vi "Numeric Control - Radio.vi"() -> ()   [LabVIEW 2015, in "Workspace.Obejct.Radio.lvlib"]
doc: "Sample numeric display item."
uses:
  Workspace.Obejct.Radio.lvlib
  <vilib>/NI Veristand/Display Template Support/Display Template Support.llb/cluster_Screen Item Settings.ctl
  <vilib>/NI Veristand/Display Template Support/Display Template Support.llb/cluster_Graph Scale Settings.ctl
  <vilib>/NI Veristand/Display Template Support/Display Template Support.llb/cluster_Graph Plot Settings.ctl
  NationalInstruments.VeriStand.SystemStorage
  <vilib>/NI Veristand/Display Template Support/Display Template Support.llb/enum_Display Template Handler Minimal To Widget Msg.ctl
  <vilib>/NI Veristand/Display Template Support/Display Template Support.llb/enum_Display Template Handler Minimal To Workspace.ctl
  Types/StateVariables.ctl
  <vilib>/NI Veristand/Execution/Workspace/WorkspaceAPI.ctl
  Types/SavedStateData.ctl
  Types/Config.ctl
  <vilib>/NI Veristand/Execution/Workspace/SystemStateEventRef.ctl
  <vilib>/NI Veristand/Execution/Workspace/Target State Info.ctl
  <vilib>/NI Veristand/Execution/Workspace/Target State.ctl
  <vilib>/NI Veristand/Execution/Workspace/SystemStateRegEventRef.ctl
  <vilib>/NI Veristand/Display Template Support/Display Template Support.llb/sub_Display Template Handler Custom.vi
  <vilib>/NI Veristand/Execution/Workspace/NI VeriStand - Set Single Channel Value.vi
  <vilib>/NI Veristand/Execution/Workspace/NI VeriStand - Get Single Channel Value.vi
  <vilib>/NI Veristand/Execution/Workspace/NI_VS Workspace ExecutionAPI.lvlib
  NationalInstruments.VeriStand.ClientAPI
panel:
  in  "NIVS.Gateway IP Address":string
  in  "Listbox":i32(listbox) caption="Channel"
  in  "NIVS.System Definition Root":refnum<k24>
  in  "Item.Data":T1
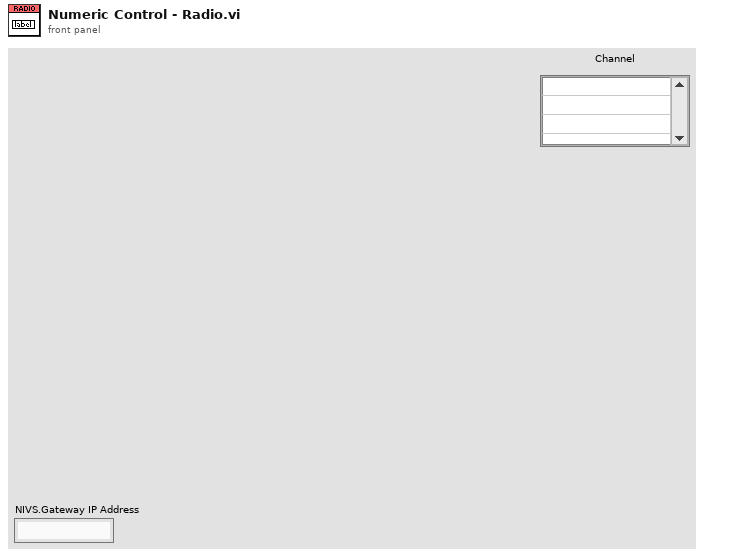
[diagram p1: front panel]
types:
  T1 = typedef "cluster_Screen Item Settings.ctl" = cluster{"Template VI":string, "Position X":i32, "Position Y":i32, "Custom":string, "Show Title Bar":bool, "ID":i32, "Always On Top":bool, "Allow Resize":bool, "Allow Minimize":bool, "Allow Close":bool, "Size to Screen":bool, "Screen.ID":i32, "State":enum16{"Normal", "New"}, "Title":string, "Window Bounds":cluster{"[0]":i16, "[1]":i16, "[2]":i16, "[3]":i16}, "Channel Ref":u64, "Unit":string, "Default Units?":bool, "Flash Limit?":bool, "Color 1":u32, "Color 2":u32, "Color 3":u32, "Color 4":u32, "Bck Color":u32, "Fore Color":u32, "Limit 1":dbl, "Limit 2":dbl, "Limit 3":dbl, "Limit 4":dbl, "Limit Mode 1":i32, "Limit Mode 2":i32, "Limit Mode 3":i32, "Limit Mode 4":i32, "Scale Precision":i32, "Scale Min":dbl, "Scale Max":dbl, "Format":i32, "Precision":i32, "Background Type":i32, "IDs":i32[], "Units":string[], "Labels":string[], "Scale Factor":dbl, "Scale Offset":dbl, "YScale Index":u32[], "XScale":T2, "YScales":T2[], "Plots":T3[], "Update Period":dbl, "History Length":dbl, "My.Ref":refnum<vi>, "Is Control?":bool, "Channel Paths":string[], "Custom Data":variant}
  T2 = typedef "cluster_Graph Scale Settings.ctl" = cluster{"Format":u8, "Precision":u8, "Fit":u8, "Label":string, "Use Default Label":bool, "Label Visible":bool, "Min":dbl, "Max":dbl}
  T3 = typedef "cluster_Graph Plot Settings.ctl" = cluster{"Bar Style":u8, "Fill To":i16, "Fill/PtColor":u32, "Line Style":u8, "Line Width":u8, "Color":u32, "Interp":u8, "Point Style":u8}
  T4 = typedef "Workspace.Obejct.Radio.lvlib/StateVariables.ctl" = cluster{"NIVS.CachedDataRef":refnum<user-event>, "NIVS.LaunchRef":refnum<user-event>, "NIVS.SysDefRoot":refnum<k24>, "NIVS.Workspace":T5, "NIVS.CachedData":T6, "NIVS.SystemStateRefs":T8, "NIVS.UserEventRefs":cluster{"SystemChangeEventRef":T9, "Event Registration Refnum":refnum<event-registration>}, "Workspace.Connected?":bool, "Workspace.ChannelFound?":bool, "UI.Listbox":refnum<vi>, "VS.DisplayFilter":u8, "Force?":bool}
  T5 = typedef "NI_VS Workspace ExecutionAPI.lvlib/WorkspaceAPI.ctl" = refnum<k24>
  T6 = typedef "Workspace.Obejct.Radio.lvlib/SavedStateData.ctl" = cluster{"Name":string, "Node Path":string, "Caption":string, "List":T7}
  T7 = typedef "Workspace.Obejct.Radio.lvlib/Config.ctl" = cluster{"AutoUpdate":bool, "Names":string[], "Values":dbl[], "Symbols":i32[]}
  T8 = typedef "NI_VS Workspace ExecutionAPI.lvlib/SystemStateEventRef.ctl" = cluster{"CustDatRef":refnum<user-event>, "EvtRef":refnum<k27>, "Target State User Event":refnum<user-event>}
  T9 = typedef "NI_VS Workspace ExecutionAPI.lvlib/SystemStateRegEventRef.ctl" = refnum<event-registration>
  T10 = typedef "enum_Display Template Handler Minimal To Workspace.ctl" = cluster{"Operation":enum16{"SetCustomData", "DeleteItem"}, "Data":variant}
  T11 = typedef "enum_Display Template Handler Minimal To Widget Msg.ctl" = enum16{"Stop", "LaunchConfigDialog"}
  T12 = typedef "NI_VS Workspace ExecutionAPI.lvlib/SystemState.ctl" = u8
  T13 = cluster{"SystemChangeEventRef":T9, "Event Registration Refnum":refnum<event-registration>}
  T14 = typedef "NI_VS UI Single Node Browser.lvlib/Node Ref.ctl" = refnum<k24>
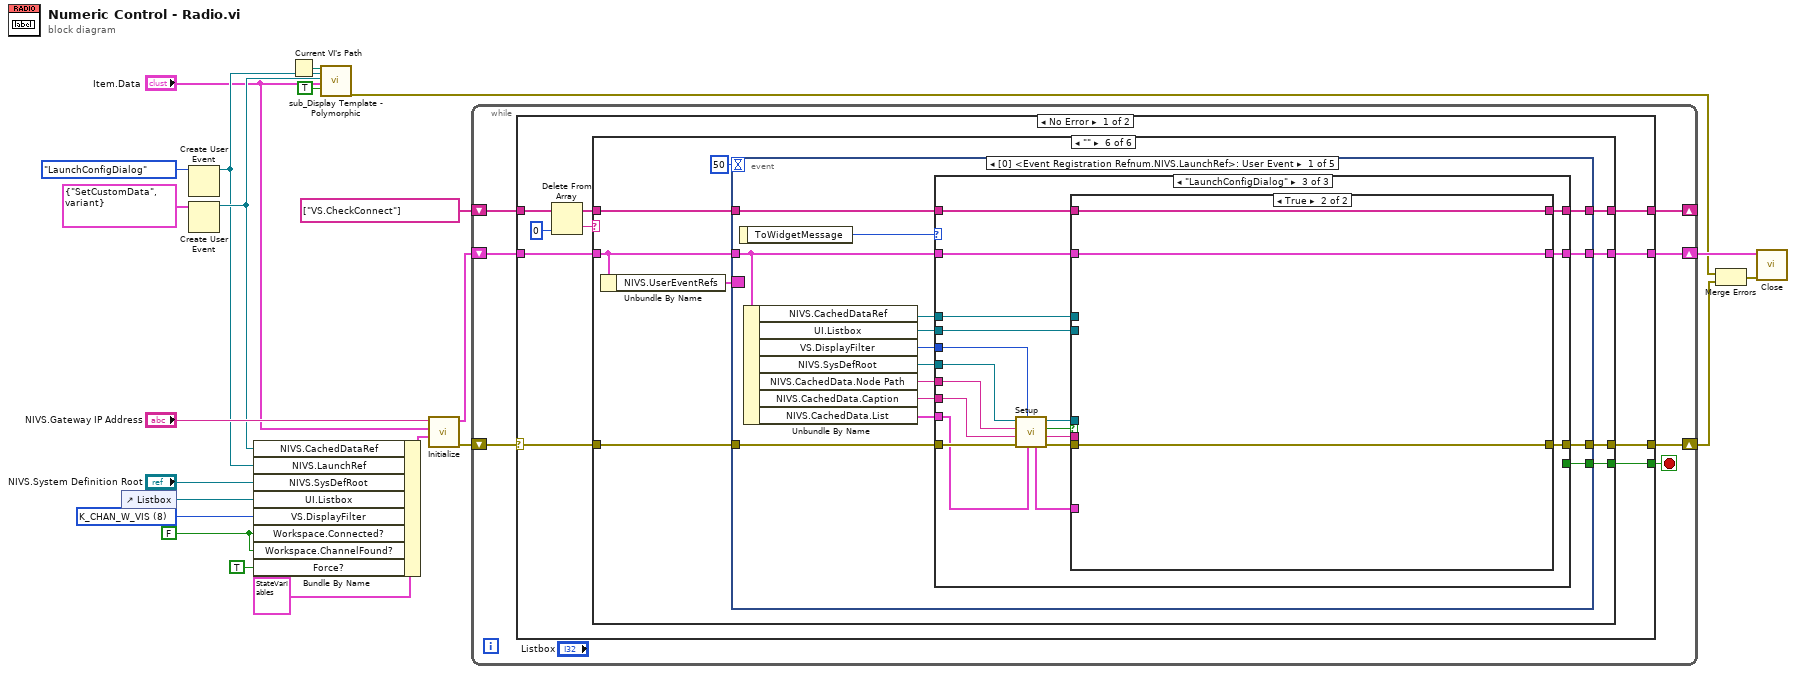
[diagram p0: block diagram]
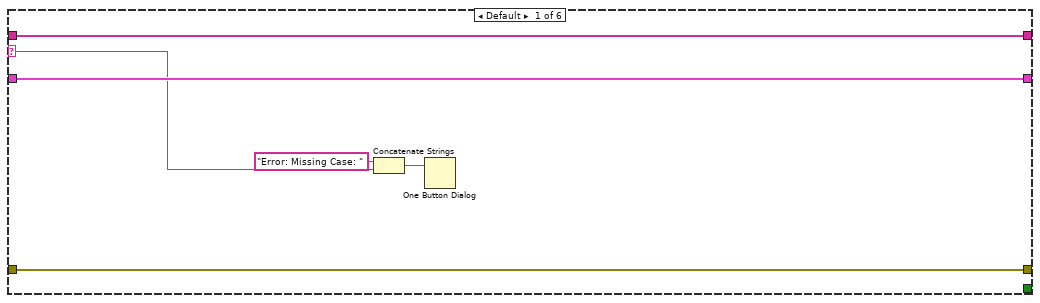
[diagram p2: hidden frame]
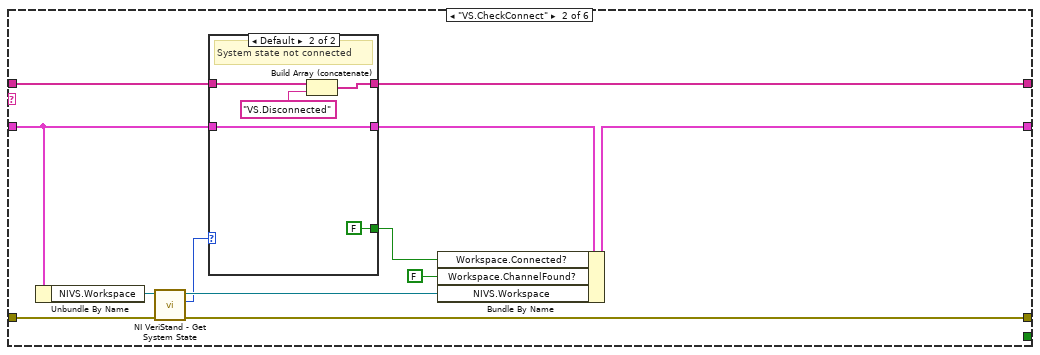
[diagram p3: hidden frame]
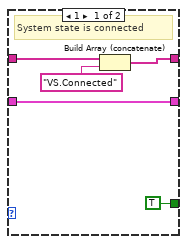
[diagram p4: hidden frame]
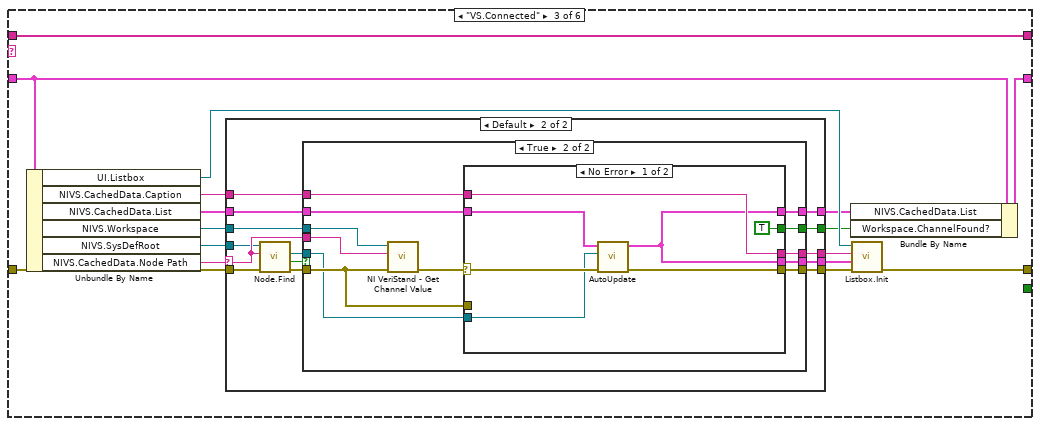
[diagram p5: hidden frame]
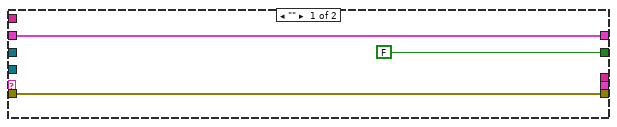
[diagram p6: hidden frame]
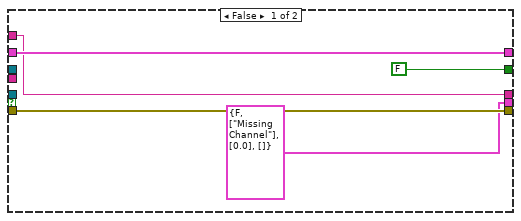
[diagram p7: hidden frame]
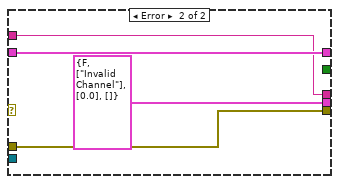
[diagram p8: hidden frame]
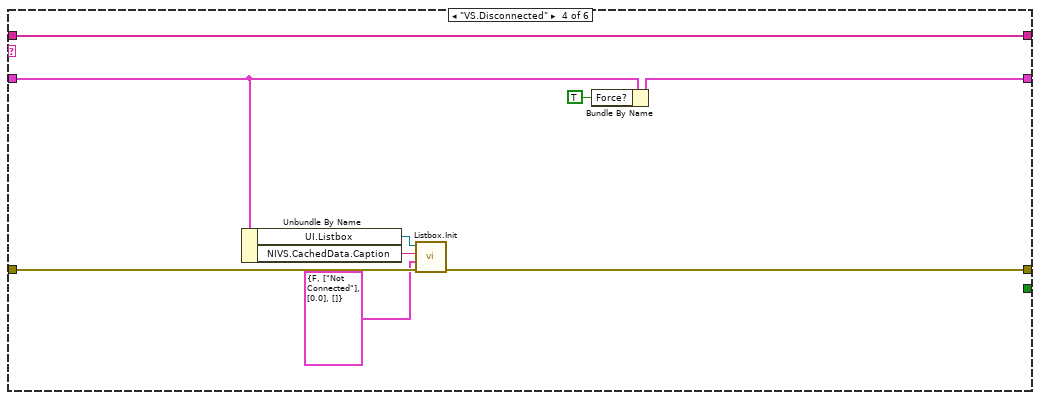
[diagram p9: hidden frame]
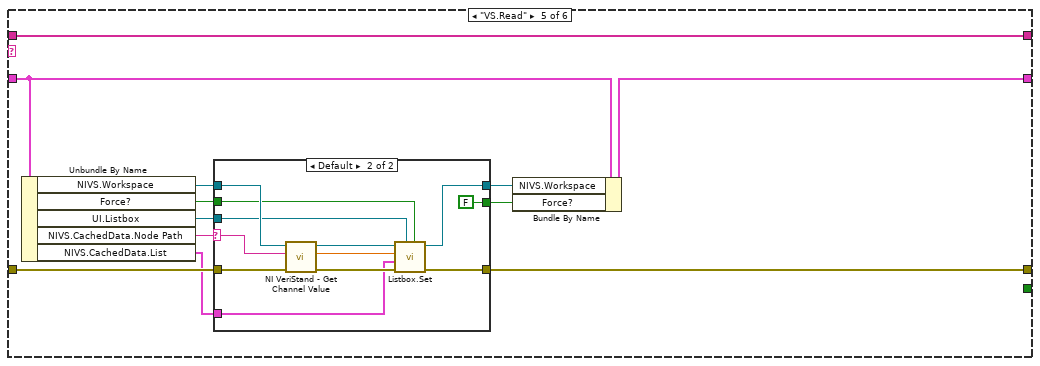
[diagram p10: hidden frame]
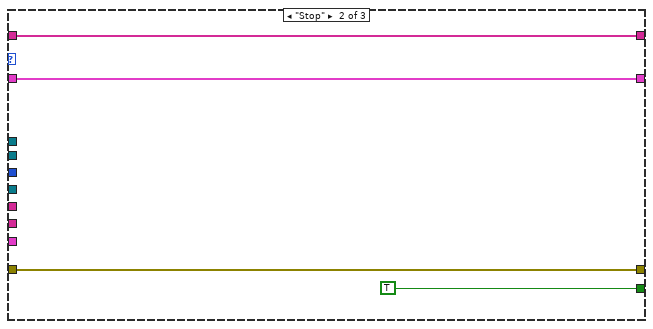
[diagram p13: hidden frame]
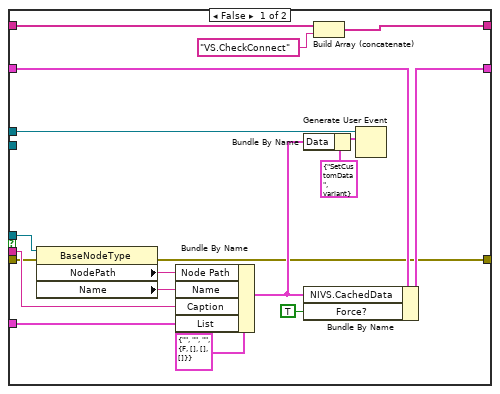
[diagram p14: hidden frame]
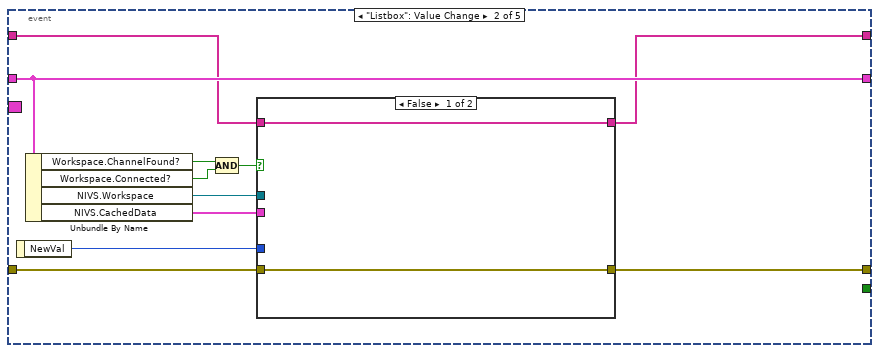
[diagram p15: hidden frame]
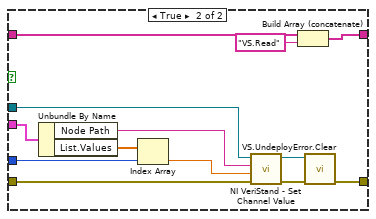
[diagram p16: hidden frame]
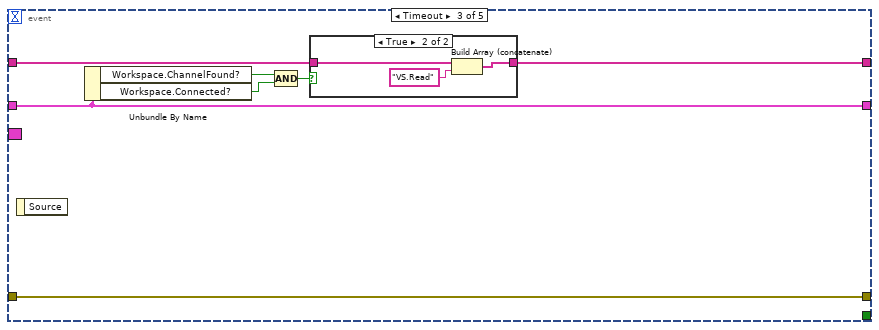
[diagram p17: hidden frame]
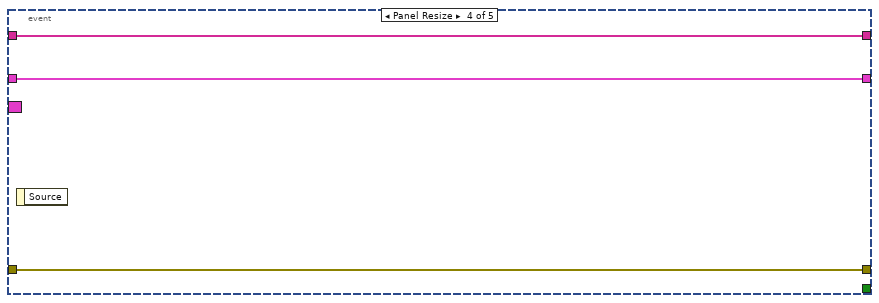
[diagram p19: hidden frame]
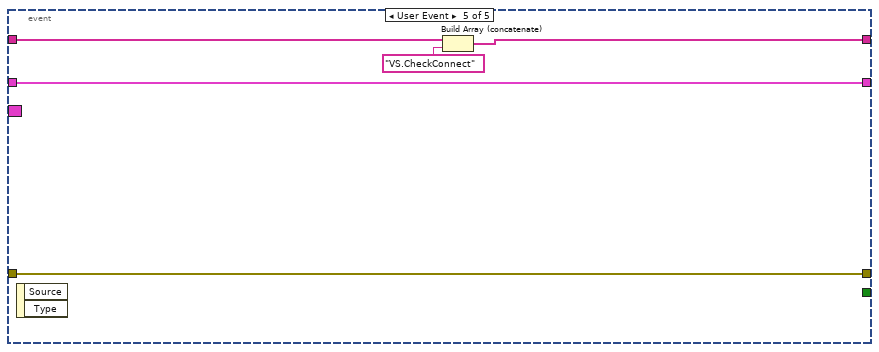
[diagram p20: hidden frame]
diagram:
  w2 = FALSE ("Workspace.Connected?")
  w3 = u8 8 items=["K_CHAN_R", "K_CHAN_W", "K_CHAN_RW", "K_CHAN_VOLT", "K_CHAN_FAULT", "K_ALL", "K_CUSTOM", "K_CHAN_R_VIS", "K_CHAN_W_VIS", "K_CHAN_RW_VIS", "K_CHAN_VOLT_VIS", "K_CHAN_FAULT_VIS"] ("DisplayFilter")
  n1 = control-ref of="Listbox"() -> (w5:refnum<vi>)
  n2 = Create User Event(user event datatype=enum_Display_Template_Handler_Minimal_To_Widget_Msg."LaunchConfigDialog" ("ToWidgetMessage")) -> (user event=w12:refnum<user-event>)  [unwired: 1 in, 1 out]
  n3 = Create User Event(user event datatype=T10 {"Operation"=enum."SetCustomData", "Data"=variant} ("Data")) -> (user event=w13:refnum<user-event>)  [unwired: 1 in, 1 out]
  n4 = Bundle By Name(cluster=T4 {"NIVS.CachedDataRef"=refnum, "NIVS.LaunchRef"=refnum, "NIVS.SysDefRoot"=refnum, "NIVS.Workspace"=refnum, "NIVS.CachedData"={"Name"="", "Node Path"="", "Caption"="", "List"={"AutoUpdate"=FALSE, "Names"=[], "Values"=[], "Symbols"=[]}}, "NIVS.SystemStateRefs"={"CustDatRef"=refnum, "EvtRef"=refnum, "Target State User Event"=refnum}, "NIVS.UserEventRefs"={"SystemChangeEventRef"=refnum, "Event Registration Refnum"=refnum}, "Workspace.Connected?"=FALSE, "Workspace.ChannelFound?"=FALSE, "UI.Listbox"=refnum, "VS.DisplayFilter"=7, "Force?"=FALSE} ("State Variables in"), "NIVS.CachedDataRef"=w13, "NIVS.LaunchRef"=w12, "NIVS.SysDefRoot"="NIVS.System Definition Root", "UI.Listbox"=w5, "VS.DisplayFilter"=w3, "Workspace.Connected?"=w2, "Workspace.ChannelFound?"=w2, "Force?"=TRUE) -> (w16:T4)
  n5 = Current VI's Path() -> (path=w20:path)
  n6 = call-poly <vilib>:"sub_Display Template - Polymorphic.vi"("Parent.Path"=w20, "ToWidgetEvent"=w12, "ToWorkspace"=w13, "Item.Data"="Item.Data", "Resizable"=TRUE) -> ("error out"=w10:errorcluster)  [unwired: 1 in, 13 out]
  n7 = call "Initialize.vi"("State Variables in"=w16, "Item.Data"="Item.Data", "NIVS.Gateway IP Address"="NIVS.Gateway IP Address") -> ("error out"=w17:errorcluster, "State Variables in"=w15:T4)  [unwired: 7 in]
  n8 = while {
    shift-right: [w28] -> w11
    shift-left: w17 -> [w25]
    shift-right: [w26] -> w14
    shift-left: w15 -> [w27]
    shift-right: [w23] -> _
    shift-left: string[] ["VS.CheckConnect"] -> [w24]
    stop <- w29 stop-if-true
    n9 = case shown="No Error" w25 {
      selector: w25 -> [w35 w281]
      tunnel: [w39 _] -> w29
      tunnel: [w38 w280] -> w28
      tunnel: w27 -> [w37 w284]
      tunnel: [w36 w284] -> w26
      tunnel: w24 -> [w33 w283]
      tunnel: [w30 w283] -> w23
      frame No Error {
        n10 = Delete From Array(array=w33, index=0) -> (deleted portion=w32:string, array with subset deleted=w31:string[])  [unwired: 1 in]
        n11 = case shown="\"\"" w32 {
          selector: w32 -> [w42 _ _ _ _ _]
          tunnel: [_ _ _ _ _ w173] -> w39
          tunnel: [w44 w50 w82 w135 w145 w172] -> w38
          tunnel: w37 -> [w45 w52 w70 w130 w143 w170]
          tunnel: [w45 w49 w71 w129 w142 w169] -> w36
          tunnel: w35 -> [w44 w51 w80 w136 w146 w168]
          tunnel: w31 -> [w43 w48 w83 w137 w149 w166]
          tunnel: [w43 w47 w83 w137 w149 w167] -> w30
          frame Default {
            n12 = Concatenate Strings("Error: Missing Case: " ("string"), w42) -> (w41:string)
            n13 = One Button Dialog(message=w41) -> ()  [unwired: 1 in, 1 out]
          }
          frame "VS.CheckConnect" {
            n14 = Unbundle By Name(w52) -> ("NIVS.Workspace"=w56:T5)
            n15 = call <vilib>:"NI VeriStand - Get System State.vi"("error in (no error)"=w51, "WorkspaceManager in"=w56) -> ("error out"=w50:errorcluster, "System State"=w53:T12, "WorkspaceManager  out"=w57:T5)  [unwired: 5 in, 2 out]
            n16 = case shown="Default" w53 {
              tunnel: [w62 w67] -> w47
              tunnel: [w60 w65] -> w54
              tunnel: w52 -> [w60 w65]
              tunnel: [TRUE FALSE] -> w55
              tunnel: w48 -> [w58 w63]
              frame 1 {
                # "System state is connected"
                n17 = Build Array (concatenate)(w58, "VS.Connected") -> (w62:string[])
              }
              frame Default {
                # "System state not connected"
                n18 = Build Array (concatenate)(w63, "VS.Disconnected") -> (w67:string[])
              }
            }
            n19 = Bundle By Name(cluster=w54, "Workspace.Connected?"=w55, "Workspace.ChannelFound?"=FALSE ("Workspace.Connected?"), "NIVS.Workspace"=w57) -> (w49:T4)
          }
          frame "VS.Connected" {
            n20 = Unbundle By Name(w70) -> ("UI.Listbox"=w81:refnum<vi>, "NIVS.CachedData.Caption"=w74:string, "NIVS.CachedData.List"=w76:T7, "NIVS.Workspace"=w78:T5, "NIVS.SysDefRoot"=w69:refnum<k24>, "NIVS.CachedData.Node Path"=w73:string)
            n21 = case shown="Default" w73 {
              selector: w73 -> [_ w92]
              tunnel: w80 -> [w86 w94]
              tunnel: [w86 w89] -> w79
              tunnel: w78 -> [_ w100]
              tunnel: [_ w97] -> w77
              tunnel: w76 -> [w84 w96]
              tunnel: [_ w99] -> w75
              tunnel: w74 -> [_ w98]
              tunnel: [FALSE w95] -> w72
              tunnel: w69 -> [_ w91]
              tunnel: [w84 w88] -> w68
              frame "" {
              }
              frame Default {
                n22 = call "Node.Find.vi"("error in (no error)"=w94, "nodePath"=w92, "System Def Root"=w91) -> ("error out"=w93:errorcluster, "FindNode"=w90:bool, "Node"=w87:refnum<k24>)  [unwired: 5 in, 1 out]
                n23 = case shown="True" w90 {
                  tunnel: w100 -> [_ w117]
                  tunnel: [w102 w115] -> w99
                  tunnel: w98 -> [w102 w114]
                  tunnel: [T7 {"AutoUpdate"=FALSE, "Names"=["Missing Channel"], "Values"=[0.0], "Symbols"=[]} ("List") w113] -> w97
                  tunnel: w96 -> [w103 w112]
                  tunnel: [FALSE w111] -> w95
                  tunnel: w93 -> [w105 w107]
                  tunnel: w92 -> [_ w110]
                  tunnel: [w105 w108] -> w89
                  tunnel: [w103 w109] -> w88
                  tunnel: w87 -> [_ w106]
                  frame False {
                  }
                  frame True {
                    n24 = call-poly <vilib>:"NI VeriStand - Get Channel Value.vi"("error in (no error)"=w107, "Channel"=w110, "WorkspaceManager in"=w117) -> ("error out"=w116:errorcluster)  [unwired: 6 in, 2 out]
                    n25 = case shown="No Error" w116 {
                      selector: w116 -> [w122 _]
                      tunnel: [w124 w126] -> w115
                      tunnel: w114 -> [w124 w126]
                      tunnel: [w120 T7 {"AutoUpdate"=FALSE, "Names"=["Invalid Channel"], "Values"=[0.0], "Symbols"=[]} ("List")] -> w113
                      tunnel: w112 -> [w118 w128]
                      tunnel: [TRUE _] -> w111
                      tunnel: [w120 w128] -> w109
                      tunnel: [w121 w127] -> w108
                      tunnel: w107 -> [_ w127]
                      tunnel: w106 -> [w119 _]
                      frame No Error {
                        n26 = call "AutoUpdate.vi"("error in (no error)"=w122, "Node"=w119, "List in"=w118) -> ("error out"=w121:errorcluster, "List out"=w120:T7)  [unwired: 7 in]
                      }
                      frame Error {
                      }
                    }
                  }
                }
              }
            }
            n27 = Bundle By Name(cluster=w70, "NIVS.CachedData.List"=w68, "Workspace.ChannelFound?"=w72) -> (w71:T4)
            n28 = call "Listbox.Init.vi"("error in (no error)"=w79, "Config"=w77, "Caption.Text"=w75, "Listbox"=w81) -> ("error out"=w82:errorcluster)  [unwired: 6 in, 1 out]
          }
          frame "VS.Disconnected" {
            n29 = Unbundle By Name(w130) -> ("UI.Listbox"=w134:refnum<vi>, "NIVS.CachedData.Caption"=w133:string)
            n30 = call "Listbox.Init.vi"("error in (no error)"=w136, "Config"=T7 {"AutoUpdate"=FALSE, "Names"=["Not Connected"], "Values"=[0.0], "Symbols"=[]} ("List"), "Caption.Text"=w133, "Listbox"=w134) -> ("error out"=w135:errorcluster)  [unwired: 6 in, 1 out]
            n31 = Bundle By Name(cluster=w130, "Force?"=TRUE) -> (w129:T4)
          }
          frame "VS.Read" {
            n32 = Unbundle By Name(w143) -> ("NIVS.Workspace"=w147:T5, "Force?"=w139:bool, "UI.Listbox"=w140:refnum<vi>, "NIVS.CachedData.Node Path"=w148:string, "NIVS.CachedData.List"=w141:T7)
            n33 = case shown="Default" w148 {
              selector: w148 -> [_ w163]
              tunnel: w147 -> [w152 w164]
              tunnel: [w150 w161] -> w145
              tunnel: [w152 w153] -> w144
              tunnel: w146 -> [w150 w160]
              tunnel: w141 -> [_ w159]
              tunnel: w140 -> [_ w155]
              tunnel: w139 -> [w151 w156]
              tunnel: [w151 FALSE ("Force?")] -> w138
              frame "" {
              }
              frame Default {
                n34 = call-poly <vilib>:"NI VeriStand - Get Channel Value.vi"("error in (no error)"=w160, "Channel"=w163, "WorkspaceManager in"=w164) -> ("error out"=w162:errorcluster, "Value"=w158:dbl, "WorkspaceManager out"=w154:T5)  [unwired: 6 in]
                n35 = call "Listbox.Set.vi"("Force?"=w156, "UI.Listbox"=w155, "error in (no error)"=w162, "List"=w159, "Value"=w158, "WorkspaceManager"=w154) -> ("error out"=w161:errorcluster, "WorkspaceManager out"=w153:T5)  [unwired: 4 in]
              }
            }
            n36 = Bundle By Name(cluster=w143, "NIVS.Workspace"=w144, "Force?"=w138) -> (w142:T4)
          }
          frame "" {
            n37 = Unbundle By Name(w170) -> ("NIVS.UserEventRefs"=w171:T13)
            n38 = event shown="[0] <Event Registration Refnum.NIVS.LaunchRef>: User Event" {
              selector: w171 -> [_ _ _ _ _]
              dyn-events: _ -> [_ _ _ _ _]
              timeout: 50 -> [_ _ _ _ _]
              tunnel: [w187 _ _ _ _] -> w173
              tunnel: [w186 w243 w266 w273 w276] -> w169
              tunnel: w168 -> [w181 w240 w267 w274 w275]
              tunnel: [w182 w237 w267 w274 w275] -> w172
              tunnel: w170 -> [w184 w243 w266 w273 w276]
              tunnel: [w180 w235 w264 w272 w277] -> w167
              tunnel: w166 -> [w179 w236 w265 w272 w278]
              event User Event {
                n39 = event-data() -> ("ToWidgetMessage"=w188:T11)  [unwired: 1 out]
                n40 = Unbundle By Name(w184) -> ("NIVS.CachedDataRef"=w185:refnum<user-event>, "UI.Listbox"=w175:refnum<vi>, "VS.DisplayFilter"=w174:u8, "NIVS.SysDefRoot"=w183:refnum<k24>, "NIVS.CachedData.Node Path"=w178:string, "NIVS.CachedData.Caption"=w177:string, "NIVS.CachedData.List"=w176:T7)
                n41 = case shown="\"LaunchConfigDialog\"" w188 {
                  tunnel: [_ TRUE _] -> w187
                  tunnel: w185 -> [_ _ w209]
                  tunnel: w183 -> [_ _ w205]
                  tunnel: [w191 w192 w207] -> w186
                  tunnel: w184 -> [w191 w192 w208]
                  tunnel: [w190 w194 w200] -> w182
                  tunnel: w181 -> [w190 w194 w206]
                  tunnel: [w189 w193 w196] -> w180
                  tunnel: w179 -> [w189 w193 w197]
                  tunnel: w178 -> [_ _ w204]
                  tunnel: w177 -> [_ _ w203]
                  tunnel: w176 -> [_ _ w202]
                  tunnel: w175 -> [_ _ w201]
                  tunnel: w174 -> [_ _ w198]
                  frame Default {
                  }
                  frame "Stop" {
                  }
                  frame "LaunchConfigDialog" {
                    n42 = call "Setup.vi"("Config in"=w202, "DisplayFilter"=w198, "error in (no error)"=w206, "Caption"=w203, "nodePath"=w204, "NIVS.System Definition Root"=w205) -> ("error out"=w199:errorcluster, "Caption out"=w211:string, "Cancel?"=w213:bool, "Selected Item"=w212:T14, "List out"=w210:T7)  [unwired: 1 in]
                    n43 = case shown="True" w213 {
                      tunnel: w209 -> [w231 _]
                      tunnel: w212 -> [w228 _]
                      tunnel: [w221 w234] -> w207
                      tunnel: w208 -> [w222 w234]
                      tunnel: w211 -> [w225 _]
                      tunnel: w210 -> [w224 _]
                      tunnel: w201 -> [_ _]
                      tunnel: [w218 w233] -> w200
                      tunnel: w199 -> [w219 w233]
                      tunnel: w197 -> [w215 w232]
                      tunnel: [w214 w232] -> w196
                      frame False {
                        n44 = property class="BaseNodeType"(reference=w228, error in=w219) -> (error out=w218:errorcluster, "NodePath"=w227:string, "Name"=w226:string)  [unwired: 1 out]
                        n45 = Bundle By Name(cluster=T6 {"Name"="", "Node Path"="", "Caption"="", "List"={"AutoUpdate"=FALSE, "Names"=[], "Values"=[], "Symbols"=[]}} ("Cluster"), "Node Path"=w227, "Name"=w226, "Caption"=w225, "List"=w224) -> (w220:T6)
                        n46 = Bundle By Name(cluster=T10 {"Operation"=enum."SetCustomData", "Data"=variant} ("event data"), "Data"=w220) -> (w229:T10)
                        n47 = Bundle By Name(cluster=w222, "NIVS.CachedData"=w220, "Force?"=TRUE) -> (w221:T4)
                        n48 = Build Array (concatenate)(w215, "VS.CheckConnect") -> (w214:string[])
                        n49 = Generate User Event(user event=w231, event data cluster=w229) -> ()  [unwired: 2 in, 2 out]
                      }
                      frame True {
                      }
                    }
                  }
                }
              }
              event "Listbox": Value Change {
                n50 = event-data() -> ("NewVal"=w238:i32)  [unwired: 1 out]
                n51 = Unbundle By Name(w243) -> ("Workspace.ChannelFound?"=w244:bool, "Workspace.Connected?"=w245:bool, "NIVS.Workspace"=w241:T5, "NIVS.CachedData"=w239:T6)
                n52 = Compound Arithmetic op=AND(w244, w245) -> (w242:bool)
                n53 = case shown="False" w242 {
                  tunnel: w241 -> [_ w259]
                  tunnel: w240 -> [w247 w260]
                  tunnel: w239 -> [_ w258]
                  tunnel: w238 -> [_ w249]
                  tunnel: [w247 w253] -> w237
                  tunnel: w236 -> [w246 w257]
                  tunnel: [w246 w255] -> w235
                  frame False {
                  }
                  frame True {
                    n54 = Unbundle By Name(w258) -> ("Node Path"=w251:string, "List.Values"=w250:dbl[])
                    n55 = Index Array(array=w250, index=w249) -> (element=w248:dbl)
                    n56 = call-poly <vilib>:"NI VeriStand - Set Channel Value.vi"("error in (no error)"=w260, "Value"=w248, "Channel"=w251, "WorkspaceManager in"=w259) -> ("error out"=w254:errorcluster, "WorkspaceManager out"=w252:T5)  [unwired: 6 in]
                    n57 = Build Array (concatenate)(w257, "VS.Read") -> (w255:string[])
                    n58 = call "VS.UndeployError.Clear.vi"("error in (no error)"=w254, "WorkspaceManager in"=w252) -> ("error out"=w253:errorcluster)  [unwired: 8 in, 1 out]
                  }
                }
              }
              event Timeout {
                n59 = event-data() -> ()  [unwired: 2 out]
                n60 = Unbundle By Name(w266) -> ("Workspace.ChannelFound?"=w262:bool, "Workspace.Connected?"=w263:bool)
                n61 = Compound Arithmetic op=AND(w262, w263) -> (w261:bool)
                n62 = case shown="True" w261 {
                  tunnel: w265 -> [w268 w271]
                  tunnel: [w268 w269] -> w264
                  frame False {
                  }
                  frame True {
                    n63 = Build Array (concatenate)(w271, "VS.Read") -> (w269:string[])
                  }
                }
              }
              event Panel Resize {
                n64 = event-data() -> ()  [unwired: 2 out]
              }
              event User Event {
                n65 = event-data() -> ()  [unwired: 3 out]
                n66 = Build Array (concatenate)(w278, "VS.CheckConnect") -> (w277:string[])
              }
            }
          }
        }
      }
      frame Error {
        n67 = call <vilib>:"Simple Error Handler.vi"("error in (no error)"=w281) -> ("error out"=w282:errorcluster)  [unwired: 4 in, 4 out]
        n68 = call <vilib>:"Clear Errors.vi"("error in (no error)"=w282) -> ("error out"=w280:errorcluster)  [unwired: 5 in, 1 out]
      }
    }
  }
  n69 = Merge Errors(w10, w11) -> (w9:errorcluster)
  n70 = call "Close.vi"("error in (no error)"=w9, "State Variables in"=w14) -> ()  [unwired: 10 in]
